vi "laser tuning derivative.vi"(8 "lower limit":dbl=3.7, 9 "upper limit":dbl=3.7, 10 "laser task in":refnum<k21>, 11 "germanium task in":refnum<k21>) -> (1 "c8 voltage":dbl, 2 "laser task out":refnum<k21>, 3 "germanium task out":refnum<k21>)   [LabVIEW 2018]
uses:
  <vilib>/DAQmx/write.llb/DAQmx Write (Analog DBL 1Chan 1Samp).vi
  0a1fad13-b885-4eab-b2d2-ceeba4e32cbd.vi
  <vilib>/DAQmx/read.llb/DAQmx Read (Analog DBL 1Chan 1Samp).vi
  <vilib>/Analysis/baseanly.llb/Mean (DBL).vi
  <vilib>/DAQmx/miscellaneous.llb/DAQmx Fill In Error Info.vi
  <vilib>/ptbypt/NI_PtbyPt.lvlib
  <vilib>/Analysis/NI_AALBase.lvlib
panel:
  out "Derivative":dbl(graph)
  out "Average":dbl(graph)
  out "current voltage":dbl
  out "diode voltage":dbl
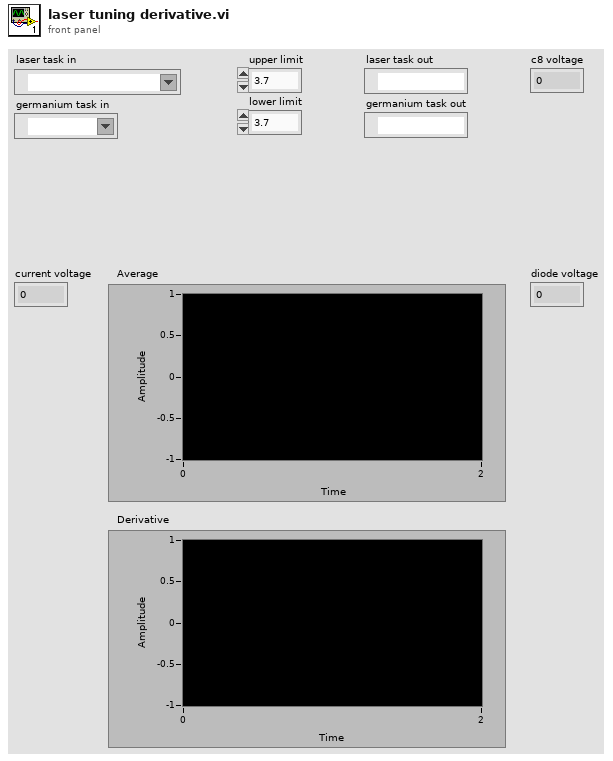
[diagram p1: front panel]
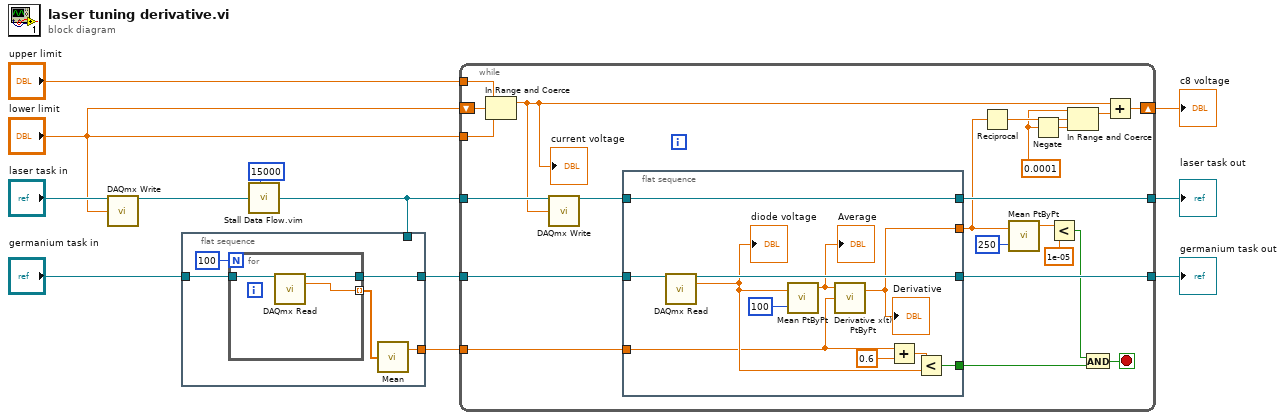
[diagram p0: block diagram]
diagram:
  n1 = call-poly <vilib>:"DAQmx Write.vi"("task/channels in"="laser task in", "data"="lower limit") -> ("task out"=w12:refnum<k21>)  [unwired: 11 in, 2 out]
  n2 = flat-sequence {
    tunnel: "germanium task in" -> [w17]
    tunnel: [w16] -> w3
    tunnel: [w13] -> w1
    tunnel: w2 -> [_]
    frame #0 {
      n3 = for {
        N: 100 -> [_]
        tunnel: [w18] -> w14 mode=indexing
        tunnel: w17 -> [w20]
        tunnel: [w19] -> w16
        n4 = call-poly <vilib>:"DAQmx Read.vi"("task/channels in"=w20) -> ("task out"=w19:refnum<k21>, "data"=w18:dbl)  [unwired: 12 in, 1 out]
      }
      n5 = call-poly <vilib>:"Mean.vi"("X"=w14) -> ("mean"=w13:dbl)  [unwired: 1 out]
    }
  }
  n6 = call "Stall Data Flow.vim"("value in"=w12, "milliseconds to wait"=u32 15000) -> ("value out"=w2:refnum<k21>)  [unwired: 1 out]
  n7 = while {
    shift-right: [w39] -> w7
    shift-left: "lower limit" -> [w38]
    tunnel: "upper limit" -> [w32]
    tunnel: "lower limit" -> [w31]
    tunnel: w3 -> [w40]
    tunnel: [w41] -> w8
    tunnel: w1 -> [w28]
    tunnel: w2 -> [w42]
    tunnel: [w29] -> w9
    stop <- w25 stop-if-true
    w34 = 0.0001 ("limit")
    n8 = In Range and Coerce(upper limit=w32, x=w38, lower limit=w31) -> (coerced(x)=w37:dbl)  [unwired: 1 out]
    "current voltage" <- w37
    n9 = call-poly <vilib>:"DAQmx Write.vi"("task/channels in"=w42, "data"=w37) -> ("task out"=w30:refnum<k21>)  [unwired: 11 in, 2 out]
    n10 = flat-sequence {
      tunnel: [w53] -> w41
      tunnel: w40 -> [w52]
      tunnel: w30 -> [w50]
      tunnel: [w50] -> w29
      tunnel: w28 -> [w44]
      tunnel: [w46] -> w21
      tunnel: [w45] -> w26
      frame #0 {
        n11 = call-poly <vilib>:"DAQmx Read.vi"("task/channels in"=w52) -> ("task out"=w53:refnum<k21>, "data"=w48:dbl)  [unwired: 12 in, 1 out]
        "diode voltage" <- w48
        n12 = call <vilib>:"Mean PtByPt.vi"("x"=w48, "sample length"=100) -> ("mean"=w49:dbl)  [unwired: 2 in, 1 out]
        "Average" <- w49
        n13 = call <vilib>:"Derivative x(t) PtByPt.vi"("initial condition"=w44, "x"=w49) -> ("dx/dt"=w45:dbl)  [unwired: 2 in, 1 out]
        "Derivative" <- w45
        n14 = Add(x=w44, y=0.6) -> (x+y=w47:dbl)
        n15 = Less?(x=w47, y=w48) -> (x < y?=w46:bool)
      }
    }
    n16 = Reciprocal(x=w26) -> (1/x=w36:dbl)
    n17 = call <vilib>:"Mean PtByPt.vi"("x"=w26, "sample length"=250) -> ("mean"=w23:dbl)  [unwired: 2 in, 1 out]
    n18 = Negate(x=w34) -> (-x=w33:dbl)
    n19 = Less?(x=w23, y=1e-05 ("x")) -> (x < y?=w22:bool)
    n20 = In Range and Coerce(upper limit=w34, x=w36, lower limit=w33) -> (coerced(x)=w35:dbl)  [unwired: 1 out]
    n21 = And(x=w22, y=w21) -> (x .and. y?=w25:bool)
    n22 = Add(x=w37, y=w35) -> (x+y=w39:dbl)
  }
  "laser task out" <- w9
  "germanium task out" <- w8
  "c8 voltage" <- w7
